vi "maquina expendedora.vi"() -> ()   [LabVIEW 2015]
panel:
  out "potato chips":string
  out "chewing gum":string
  out "candy bars":string
  out "quarters":dbl
  out "dimes":dbl
  out "nickels":dbl
  out "dollar":dbl
  out "Pantalla":string
  out "Boolean":bool
  in  "chewing gum":bool
  in  "potato chips":bool
  in  "candy bars":bool
  in  "cantidad chicle":dbl min=0.0 max=10.0
  in  "cantidad papas":dbl min=0.0 max=10.0
  in  "cantidad barras":dbl min=0.0 max=10.0
  out "String 2":string
  out "String":string
  in  "Total":dbl min=0.0 max=100.0 step=0.05 format="%.3g"
  # "Tarea 1: Maquina expendedora\nRoberto Israel Nava Rodríguez"
  # "Pantalla en donde se muestran los mensajes"
  # "LED indicador de falta de efectivo"
  # "Monto que ha sido ingresado a la maquina"
  # "Indicadores del tipo de efectivo que recibe \n(requiere correr el programa una vez para mostrar)"
  # "Control de tipo y cantidad de producto"
  # "Tipo de cambio que entrega la maquina"
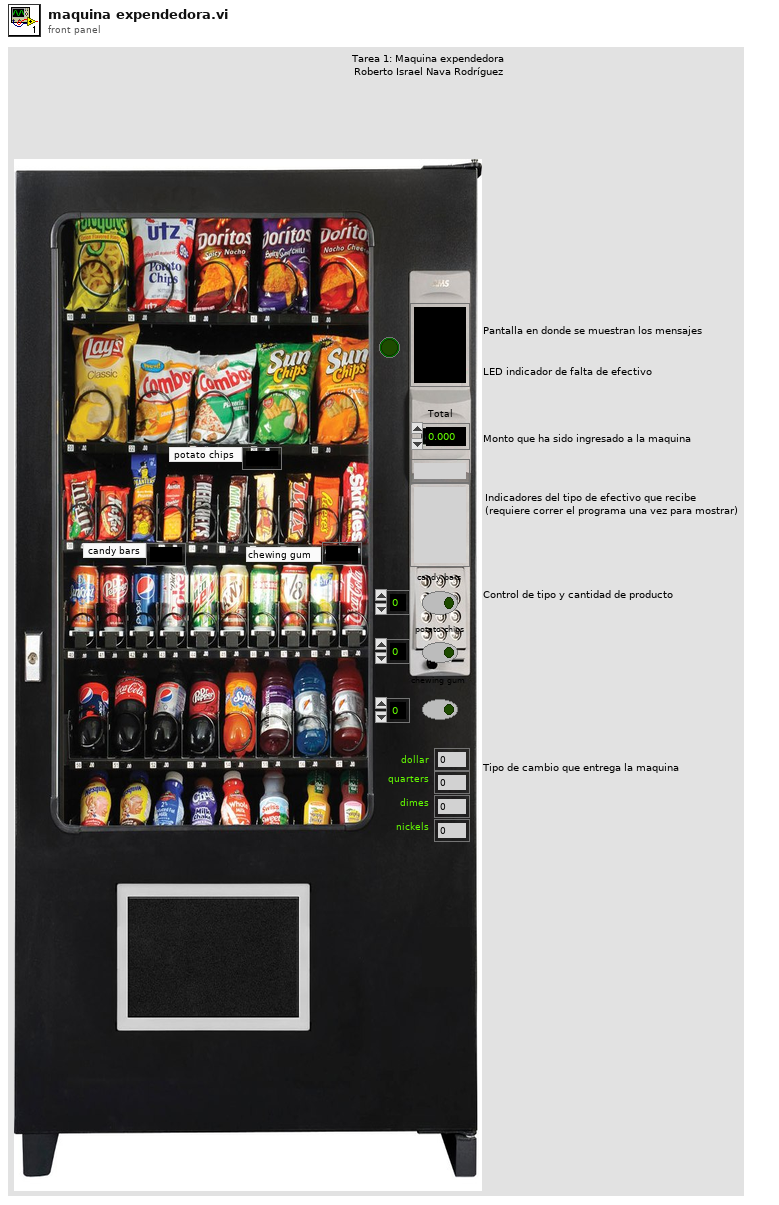
[diagram p1: front panel]
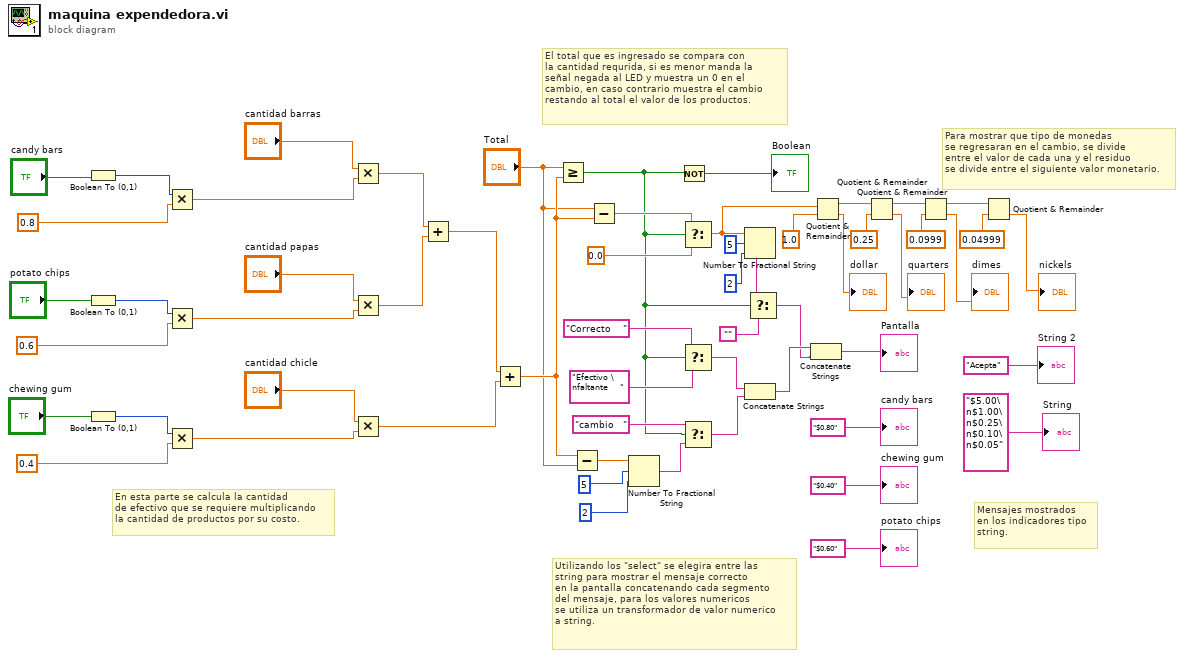
[diagram p0: block diagram]
diagram:
  # "Mensajes mostrados\nen los indicadores tipo\nstring."
  # "Para mostrar que tipo de monedas\nse regresaran en el cambio, se divide \nentre el valor de cada una y el residuo \nse divide entre el siguiente valor monetario."
  # "Utilizando los \"select\" se elegira entre las\nstring para mostrar el mensaje correcto\nen la pantalla concatenando cada segmento\ndel mensaje, para los valores numericos\nse utiliza un transformador de valor numerico\na string."
  # "El total que es ingresado se compara con\nla cantidad requrida, si es menor manda la\nseñal negada al LED y muestra un 0 en el \ncambio, en caso contrario muestra el cambio \nrestando al total el valor de los productos."
  # "En esta parte se calcula la cantidad\nde efectivo que se requiere multiplicando\nla cantidad de productos por su costo."
  n1 = Boolean To (0,1)(Boolean="candy bars") -> (0, 1=w55:i16)
  n2 = Boolean To (0,1)(Boolean="potato chips") -> (0, 1=w53:i16)
  n3 = Boolean To (0,1)(Boolean="chewing gum") -> (0, 1=w51:i16)
  n4 = Multiply(x=w55, y=0.8) -> (x*y=w49:dbl)
  n5 = Multiply(x=w53, y=0.6) -> (x*y=w46:dbl)
  n6 = Multiply(x=w51, y=0.4) -> (x*y=w44:dbl)
  n7 = Multiply(x="cantidad barras", y=w49) -> (x*y=w43:dbl)
  n8 = Multiply(x="cantidad papas", y=w46) -> (x*y=w42:dbl)
  n9 = Multiply(x="cantidad chicle", y=w44) -> (x*y=w41:dbl)
  n10 = Add(x=w43, y=w42) -> (x+y=w40:dbl)
  n11 = Add(x=w40, y=w41) -> (x+y=w34:dbl)
  n12 = Greater Or Equal?(x="Total", y=w34) -> (x >= y?=w22:bool)
  n13 = Subtract(x=w34, y="Total") -> (x-y=w27:dbl)
  n14 = Subtract(x="Total", y=w34) -> (x-y=w39:dbl)
  n15 = Number To Fractional String(number=w27, width (-)=5, precision (6)=2) -> (F-format string=w24:string)  [unwired: 1 in]
  n16 = Not(x=w22) -> (.not. x?=→"Boolean":bool)
  n17 = Select(t=w39, s=w22, f=0.0) -> (s? t:f=w15:dbl)
  n18 = Select(t="Correcto    ", s=w22, f="Efectivo \nfaltante    ") -> (s? t:f=w30:string)
  n19 = Select(t="cambio   ", s=w22, f=w24) -> (s? t:f=w29:string)
  n20 = Number To Fractional String(number=w15, width (-)=5, precision (6)=2) -> (F-format string=w20:string)  [unwired: 1 in]
  n21 = Concatenate Strings(w30, w29) -> (w18:string)
  n22 = Select(t=w20, s=w22, f="") -> (s? t:f=w17:string)
  n23 = Concatenate Strings(w18, w17) -> (→"Pantalla":string)
  n24 = Quotient & Remainder(x=w15, y=1.0) -> (x-y*floor(x/y)=w10:dbl, floor(x/y)=→"dollar":dbl)
  n25 = Quotient & Remainder(x=w10, y=0.25) -> (x-y*floor(x/y)=w9:dbl, floor(x/y)=→"quarters":dbl)
  n26 = Quotient & Remainder(x=w9, y=0.0999) -> (x-y*floor(x/y)=w8:dbl, floor(x/y)=→"dimes":dbl)
  n27 = Quotient & Remainder(x=w8, y=0.04999) -> (floor(x/y)=→"nickels":dbl)  [unwired: 1 out]
  "String" <- "$5.00\n$1.00\n$0.25\n$0.10\n$0.05"
  "String 2" <- "Acepta"
  "candy bars" <- "$0.80"
  "chewing gum" <- "$0.40"
  "potato chips" <- "$0.60"
